vi "Update Status Event.vi"() -> (3 "Update Status":refnum<user-event>)   [LabVIEW 2020]
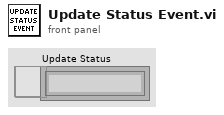
[diagram p1: front panel]
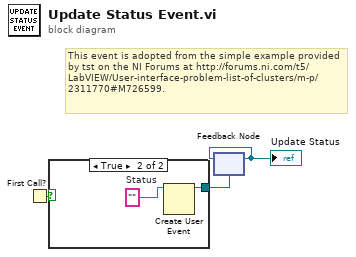
[diagram p0: block diagram]
diagram:
  # "This event is adopted from the simple example provided by tst on the NI Forums at http://forums.ni.com/t5/LabVIEW/User-interface-problem-list-of-clusters/m-p/2311770#M726599."
  n1 = First Call?() -> (First Call?: T/F=w3:bool)
  n2 = case shown="True" w3 {
    tunnel: [_ w5] -> w2
    frame False {
    }
    frame True {
      w4 = ""  # Status
      n3 = Create User Event(user event datatype=w4) -> (user event=w5:refnum<user-event>)  [unwired: 1 in, 1 out]
    }
  }
  n4 = feedback #1(w2) -> (w1:refnum<user-event>)
  "Update Status" <- w1
  n5 = feedback-in #1(w1) -> ()
